vi "Parse.vi"(8 "Error In":errorcluster, 11 "object in":refnum<class "2024_9.lvclass">) -> (0 "Error Out":errorcluster, 3 "object out":refnum<class "2024_9.lvclass">)   [LabVIEW 2023, in "2024_9.lvclass"]
uses:
  2024_9.lvclass
  2024_9.lvclass/2024_9.ctl
  <vilib>/Utility/error.llb/Trim Whitespace One-Sided.vi
panel:
  out "size(s)":i32
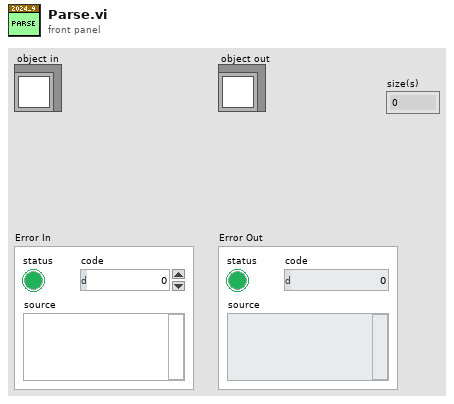
[diagram p1: front panel]
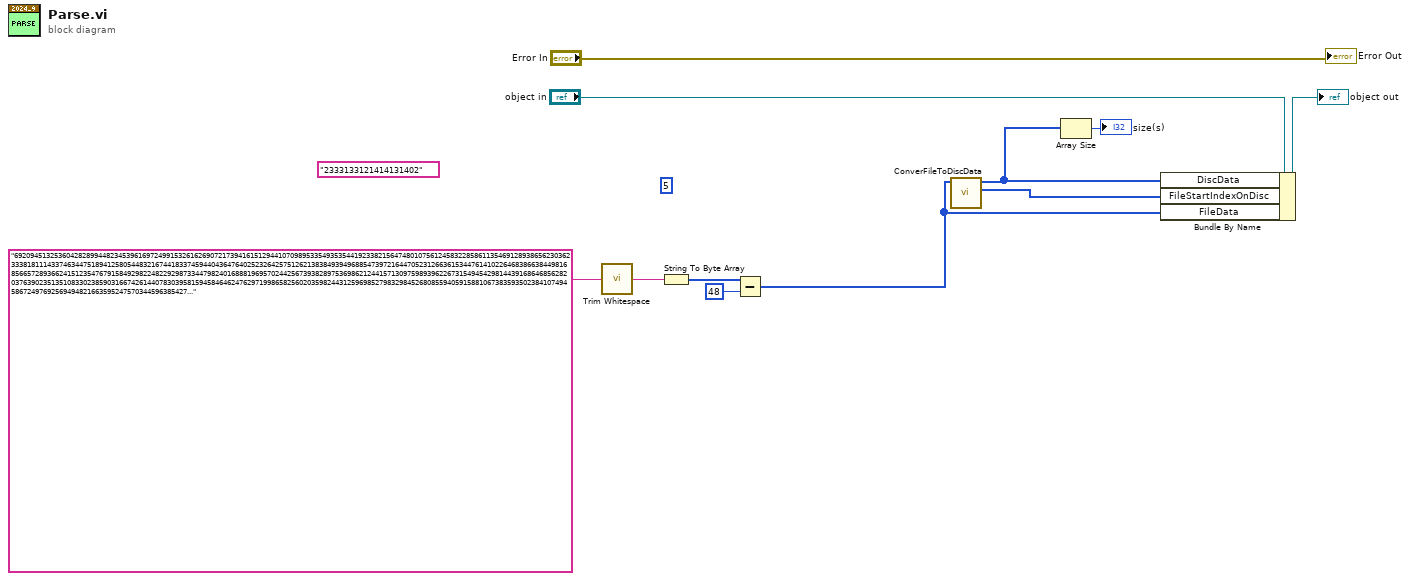
[diagram p0: block diagram]
diagram:
  (unwired) "2333133121414131402"
  (unwired) i64 5
  n1 = call <vilib>:"Trim Whitespace.vi"("string"="692094513253604282899448234539616972499153261626907217394161512944107098953354935354419233821564748010756124583228586113546912893865623036233381811143374634475189412580544832167441833745944043647640252326425751262138384939496885473972164470523126636153447614102264683866384498168566572893662415123547679158492982248229298733447982401688819695702442567393828975369862124415713097598939622673154945429814439168646856282037639023513510833023859031667426144078303958159458464624762971998658256020359824431259698527983298452680855940591588106738359350238410749458672497692569494821663595247570344596385427...") -> ("trimmed string"=w8:string)  [unwired: 1 in]
  n2 = String To Byte Array(string=w8) -> (unsigned byte array=w5:u8[])
  n3 = Subtract(x=w5, y=u8 48) -> (x-y=w4:u8[])
  n4 = call "ConverFileToDiscData.vi"("FileData"=w4) -> ("FileStartIndexOnDisc"=w2:i32[], "DiscData"=w3:i64[])  [unwired: 9 in]
  n5 = Array Size(array=w3) -> (size(s)=→"size(s)":i32)
  n6 = Bundle By Name(cluster="object in", "DiscData"=w3, "FileStartIndexOnDisc"=w2, "FileData"=w4) -> (→"object out":refnum<class "2024_9.lvclass">)
  "Error Out" <- "Error In"
